vi "Get Keithley 182 Data.vi"(8 "error in (no error)":errorcluster, 10 "data string in":string=":FETCH?", 11 "VISA Resource Name":refnum<visa-resource-name>="GPIB0::20::INSTR") -> (0 "error out":errorcluster={"status"=TRUE, "code"=-1073807339, "source"="VISA Read in VISA  Send Receive.vi->Get Keithley meter Data.vi"}, 1 "Returned string":string, 2 "Data":dbl format="%#_6p", 3 "VISA Resource Name Out":refnum<visa-resource-name>="GPIB0::20::INSTR")   [LabVIEW 2015]
panel:
  out "after substring":string
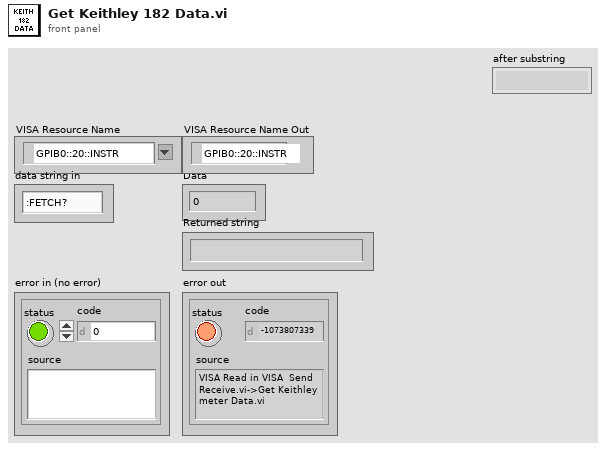
[diagram p1: front panel]
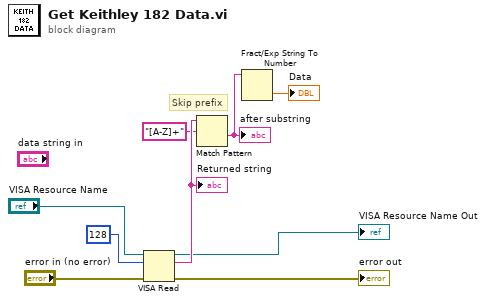
[diagram p0: block diagram]
diagram:
  # "Skip prefix"
  n1 = VISA Read(VISA resource name="VISA Resource Name", byte count=u32 128, error in (no error)="error in (no error)") -> (VISA resource name out=→"VISA Resource Name Out":refnum<visa-resource-name>, read buffer=w5:string, error out=→"error out":errorcluster)  [unwired: 1 out]
  "Returned string" <- w5
  n2 = Match Pattern(string=w5, regular expression="[A-Z]+") -> (after substring=w4:string)  [unwired: 1 in, 3 out]
  "after substring" <- w4
  n3 = Fract/Exp String To Number(string=w4) -> (number=→"Data":dbl)  [unwired: 4 out]
